vi "password creation.vi"() -> ()   [LabVIEW 2017]
panel:
  out "s? t:f":string
  out "result":bool
  out "length":i32
  in  "password":string
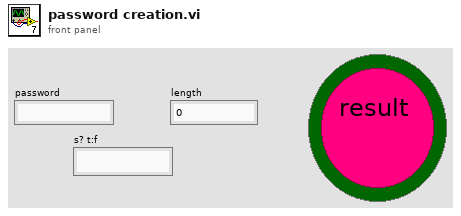
[diagram p1: front panel]
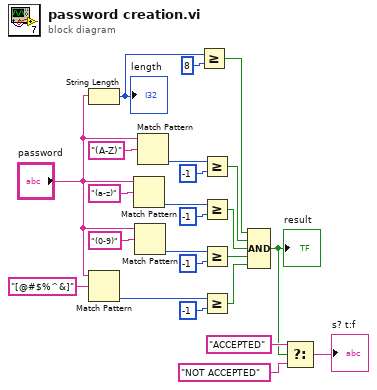
[diagram p0: block diagram]
diagram:
  n1 = String Length(string="password") -> (length=w24:i32)
  "length" <- w24
  n2 = Match Pattern(string="password", regular expression="[@#$%^&]") -> (offset past match=w13:i32)  [unwired: 1 in, 3 out]
  n3 = Match Pattern(string="password", regular expression="(a-z)") -> (offset past match=w19:i32)  [unwired: 1 in, 3 out]
  n4 = Match Pattern(string="password", regular expression="(0-9)") -> (offset past match=w14:i32)  [unwired: 1 in, 3 out]
  n5 = Match Pattern(string="password", regular expression="(A-Z)") -> (offset past match=w21:i32)  [unwired: 1 in, 3 out]
  n6 = Greater Or Equal?(x=w24, y=8) -> (x >= y?=w9:bool)
  n7 = Greater Or Equal?(x=w21, y=-1) -> (x >= y?=w8:bool)
  n8 = Greater Or Equal?(x=w19, y=-1) -> (x >= y?=w7:bool)
  n9 = Greater Or Equal?(x=w14, y=-1) -> (x >= y?=w6:bool)
  n10 = Greater Or Equal?(x=w13, y=-1) -> (x >= y?=w5:bool)
  n11 = Compound Arithmetic op=AND(w9, w8, w7, w6, w5) -> (w1:bool)
  "result" <- w1
  n12 = Select(t="ACCEPTED", s=w1, f="NOT ACCEPTED") -> (s? t:f=→"s? t:f":string)
